vi "deliver droplet.vi"(1 "channel":i8) -> ()   [LabVIEW 2023]
panel:
  out "channel":string
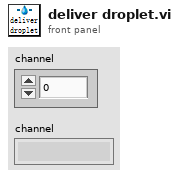
[diagram p1: front panel]
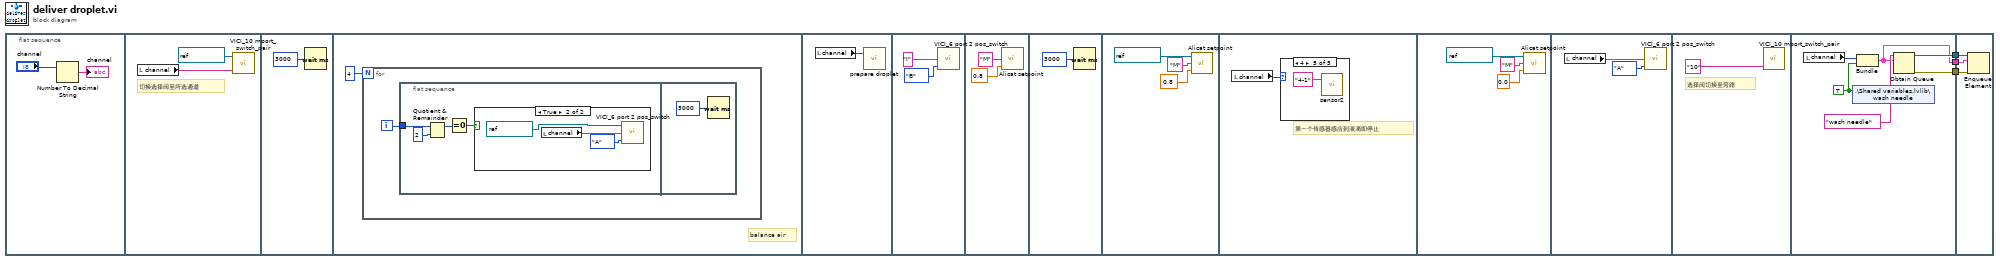
[diagram p0: block diagram]
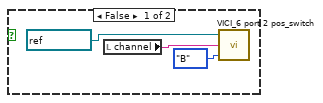
[diagram p2: hidden frame]
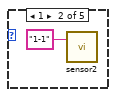
[diagram p4: hidden frame]
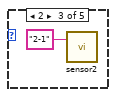
[diagram p5: hidden frame]
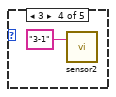
[diagram p6: hidden frame]
diagram:
  n1 = flat-sequence {
    tunnel: [w44] -> w3
    tunnel: [w43] -> w2
    tunnel: [w42] -> w1
    tunnel: w3 -> [w50]
    tunnel: w2 -> [w49]
    tunnel: w1 -> [w48]
    frame #0 {
      n2 = Number To Decimal String(number="channel") -> (decimal integer string=→"channel":string)  [unwired: 1 in]
    }
    frame #1 {
      # "切换选择阀至所选通道"
      n3 = local read "channel"() -> (w7:string)
      n4 = call "VICI_10 mport_switch_pair.vi"("Go to position"=w7, "Valve COM"=refnum<visa-resource-name> "COM8") -> ()  [unwired: 2 in, 1 out]
    }
    frame #2 {
      n5 = Wait (ms)(milliseconds to wait=u32 3000) -> ()  [unwired: 1 out]
    }
    frame #3 {
      # "balance air"
      n6 = for {
        N: 4 -> [_]
        i -> [w10]
        n7 = flat-sequence {
          tunnel: w10 -> [w14]
          frame #0 {
            n8 = Quotient & Remainder(x=w14, y=2) -> (x-y*floor(x/y)=w12:i32)  [unwired: 1 out]
            n9 = Equal To 0?(x=w12) -> (x = 0?=w11:bool)
            n10 = case shown="True" w11 {
              frame False {
                n11 = local read "channel"() -> (w15:string)
                n12 = call "VICI_6 port 2 pos_switch.vi"("Switch to position (A/B)"=enum16{"A", "B"}."B", "Valve ID"=w15, "Valve COM"=refnum<visa-resource-name> "COM8") -> ()  [unwired: 1 in, 1 out]
              }
              frame True {
                n13 = local read "channel"() -> (w18:string)
                n14 = call "VICI_6 port 2 pos_switch.vi"("Switch to position (A/B)"=enum16{"A", "B"}."A", "Valve ID"=w18, "Valve COM"=refnum<visa-resource-name> "COM8") -> ()  [unwired: 1 in, 1 out]
              }
            }
          }
          frame #1 {
            n15 = Wait (ms)(milliseconds to wait=u32 3000) -> ()  [unwired: 1 out]
          }
        }
      }
    }
    frame #4 {
      n16 = local read "channel"() -> (w22:i8)
      n17 = call "prepare droplet.vi"("channel"=w22) -> ()  [unwired: 3 in]
    }
    frame #5 {
      n18 = call "VICI_6 port 2 pos_switch.vi"("Switch to position (A/B)"=enum16{"A", "B"}."B", "Valve ID"="I") -> ()  [unwired: 2 in, 1 out]
    }
    frame #6 {
      n19 = call "Alicat setpoint.vi"("Setpoint"=0.8, "Unit ID"="M") -> ()  [unwired: 3 in]
    }
    frame #7 {
      n20 = Wait (ms)(milliseconds to wait=u32 3000) -> ()  [unwired: 1 out]
    }
    frame #8 {
      n21 = call "Alicat setpoint.vi"("Setpoint"=0.8, "Unit ID"="M", "ALICAT COM Port"=refnum<visa-resource-name> "COM5") -> ()  [unwired: 2 in]
    }
    frame #9 {
      # "第一个传感器感应到液滴即停止"
      n22 = local read "channel"() -> (w31:i8)
      n23 = case shown="4" w31 {
        frame 0, Default {
        }
        frame 1 {
          n24 = call "sensor2.vi"("Sensor"="1-1") -> ()  [unwired: 1 in, 2 out]
        }
        frame 2 {
          n25 = call "sensor2.vi"("Sensor"="2-1") -> ()  [unwired: 1 in, 2 out]
        }
        frame 3 {
          n26 = call "sensor2.vi"("Sensor"="3-1") -> ()  [unwired: 1 in, 2 out]
        }
        frame 4 {
          n27 = call "sensor2.vi"("Sensor"="4-1") -> ()  [unwired: 1 in, 2 out]
        }
      }
    }
    frame #10 {
      n28 = call "Alicat setpoint.vi"("Setpoint"=0.0, "Unit ID"="M", "ALICAT COM Port"=refnum<visa-resource-name> "COM5") -> ()  [unwired: 2 in]
    }
    frame #11 {
      n29 = local read "channel"() -> (w40:string)
      n30 = call "VICI_6 port 2 pos_switch.vi"("Switch to position (A/B)"=enum16{"A", "B"}."A", "Valve ID"=w40) -> ()  [unwired: 2 in, 1 out]
    }
    frame #12 {
      # "选择阀切换至旁路"
      n31 = call "VICI_10 mport_switch_pair.vi"("Go to position"="10") -> ()  [unwired: 3 in, 1 out]
    }
    frame #13 {
      w45 = TRUE
      n32 = local read "channel"() -> (w46:i8)
      n33 = shared-variable ".\\Shared variables.lvlib\\wash needle"(w45) -> ()  [unwired: 1 in, 1 out]
      n34 = Bundle("channel"=w46, w45) -> (w43:cluster{"channel":i8, bool})  [unwired: 1 in]
      n35 = Obtain Queue(name (unnamed)="wash needle", element data type=w43) -> (queue out=w44:refnum<queue>, error out=w42:errorcluster)  [unwired: 3 in, 1 out]
    }
    frame #14 {
      n36 = Enqueue Element(queue=w50, element=w49, error in (no error)=w48) -> ()  [unwired: 1 in, 3 out]
    }
  }
